vi "Main.vi"() -> ()   [LabVIEW 2015]
panel:
  in  "VISA资源名称":refnum<visa-resource-name>="COM20"
  in  "退出":bool
  in  "导出":bool
  in  "测试间隔（单位：分钟）":dbl
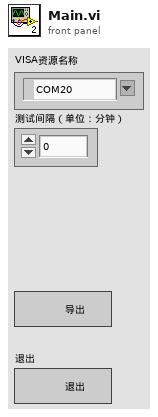
[diagram p1: front panel]
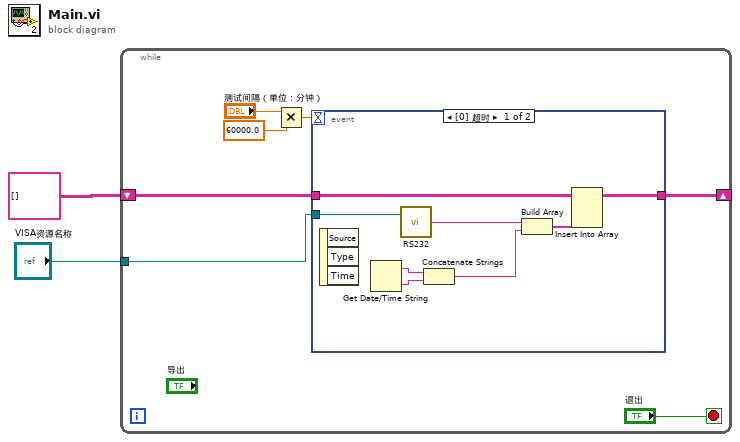
[diagram p0: block diagram]
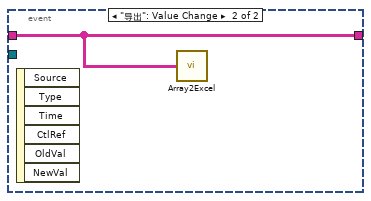
[diagram p2: hidden frame]
diagram:
  n1 = while {
    shift-right: [w4] -> _
    shift-left: string[][] [] -> [w5]
    tunnel: "VISA资源名称" -> [w3]
    stop <- "退出" stop-if-true
    n2 = Multiply(x="测试间隔（单位：分钟）", y=60000.0) -> (x*y=w7:dbl)
    n3 = event shown="[0] 超时" {
      selector: _ -> [_ _]
      dyn-events: _ -> [_ _]
      timeout: w7 -> [_ _]
      tunnel: w5 -> [w15 w18]
      tunnel: [w11 w18] -> w4
      tunnel: w3 -> [w10 _]
      event Timeout {
        n4 = event-data() -> ()  [unwired: 1 in, 3 out]
        n5 = Get Date/Time String() -> (date string=w17:string, time string=w16:string)  [unwired: 3 in]
        n6 = call "RS232.vi"("VISA资源名称"=w10) -> ("响应"=w14:string)  [unwired: 1 in]
        n7 = Concatenate Strings(w17, w16) -> (w13:string)
        n8 = Build Array(w14, w13) -> (w12:string[])
        n9 = Insert Into Array(array=w15, new element=w12) -> (w11:string[][])  [unwired: 2 in]
      }
      event "导出": Value Change {
        n10 = event-data() -> ()  [unwired: 1 in, 6 out]
        n11 = call "Array2Excel.vi"("text data"=w18) -> ()
      }
    }
  }
